vi "Global 1.vi"() -> ()   [LabVIEW 2022 SP3]
panel:
  out "path_log":path
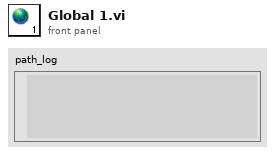
[diagram p1: front panel]
diagram:
